vi "Read 1 Waveform & Read Max Value.vi"() -> ()   [LabVIEW 2020]
uses:
  <instrlib>/LeCroy Wave Series/Public/Data/Read Single Waveform.vi
  <instrlib>/LeCroy Wave Series/LeCroy Wave Series.lvlib
panel:
  in  "Number of points (0: All points)":i32
  in  "Sparsing (0: Every point)":i32
  in  "First point (0: First point)":i32
  out "Max":waveform(dbl)(graph)
  out "Min":waveform(dbl)(graph)
  in  "Timeout (10000 ms)":u32=10000
  in  "Source (0: Channel 1)":u16(ring) items=["Channel 1", "Channel 2", "Channel 3", "Channel 4", "Memory 1", "Memory 2", "Memory 3", "Memory 4", "Function 1", "Function 2", "Function 3", "Function 4", "Function 5", "Function 6", "Function 7", "Function 8", "Other"]
  out "Waveform Data":waveform(dbl)(graph)
  out "error out":errorcluster
  in  "error in (no error)":errorcluster
  in  "Reset? (T: Yes)":bool=TRUE
  in  "ID Query? (T: Yes)":bool=TRUE
  in  "VISA resource name":refnum<visa-resource-name>
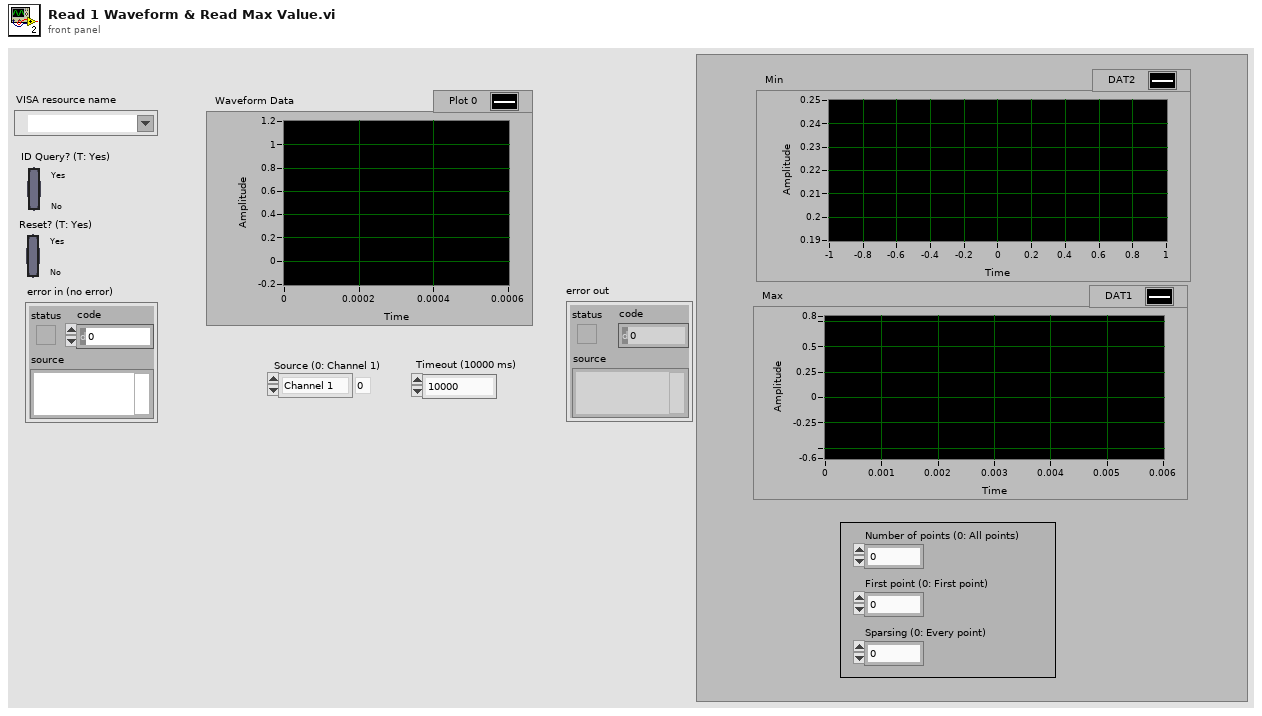
[diagram p1: front panel]
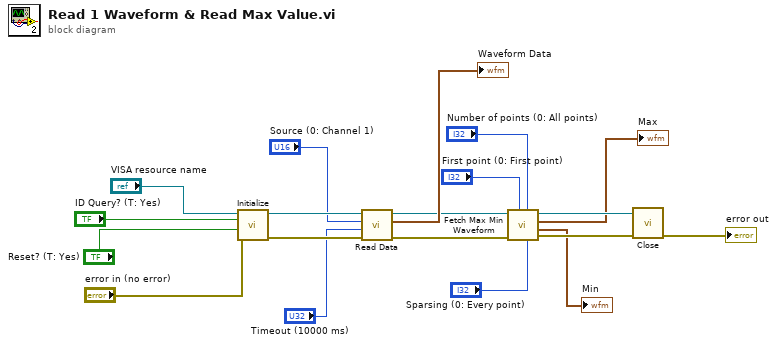
[diagram p0: block diagram]
diagram:
  n1 = call <instrlib>:"Initialize.vi"("error in (no error)"="error in (no error)", "Reset? (T: Yes)"="Reset? (T: Yes)", "ID Query? (T: Yes)"="ID Query? (T: Yes)", "VISA resource name"="VISA resource name") -> ("error out"=w13:errorcluster, "VISA resource name out"=w14:refnum<visa-resource-name>)  [unwired: 6 in]
  n2 = call-poly <instrlib>:"Read Data.vi"("error in (no error)"=w13, "Timeout (10000 ms)"="Timeout (10000 ms)", "Source (0: Channel 1)"="Source (0: Channel 1)", "VISA resource name"=w14) -> ("error out"=w6:errorcluster, "Waveform Data"=→"Waveform Data":waveform(dbl), "VISA resource name out"=w9:refnum<visa-resource-name>)  [unwired: 5 in]
  n3 = call <instrlib>:"Fetch Max Min Waveform.vi"("Sparsing (0: Every point)"="Sparsing (0: Every point)", "Number of points (0: All points)"="Number of points (0: All points)", "First point (0: First point)"="First point (0: First point)", "error in (no error)"=w6, "VISA resource name"=w9) -> ("error out"=w7:errorcluster, "Min"=→"Min":waveform(dbl), "Max"=→"Max":waveform(dbl), "VISA resource name out"=w8:refnum<visa-resource-name>)  [unwired: 3 in]
  n4 = call <instrlib>:"Close.vi"("error in (no error)"=w7, "VISA resource name"=w8) -> ("error out"=→"error out":errorcluster)  [unwired: 9 in]
